vi "fpga_set.vi"(8 "error in":errorcluster, 9 "trigger  delay":u64, 10 "num samples":u64=1000, 11 "FPGA VI Reference In":refnum<k20>) -> (0 "error out":errorcluster, 3 "FPGA VI Reference Out":refnum<k20>)   [LabVIEW 2015]
doc: "Set the FPGA to wait for a trigger and aquire a specifiecf number of samples."
uses:
  <vilib>/Utility/error.llb/Error Cluster From Error Code.vi
  <vilib>/rvi/errors/niLvFpgaAdjustHostInterfaceError.vi
  <instrlib>/_niInstr/Streaming/v1/Host/Public/Start Finite Stream.vi
  <vilib>/rvi/interface/nirviReadWriteControl/nirviReadWriteControl.xnode
  <instrlib>/_niInstr/Streaming/v1/Host/niInstr Streaming v1 Host.lvlib
  NiFpgaLv.dll
  <vilib>/rvi/interface/Simulation/niFpgaSimulationCallBeginRW.vi
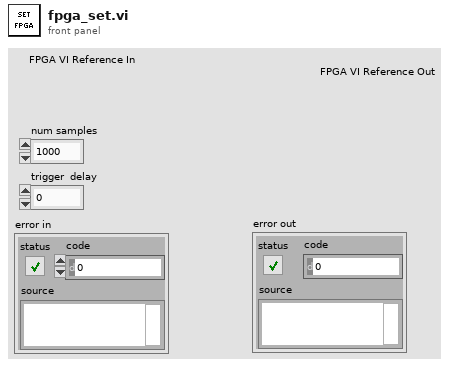
[diagram p1: front panel]
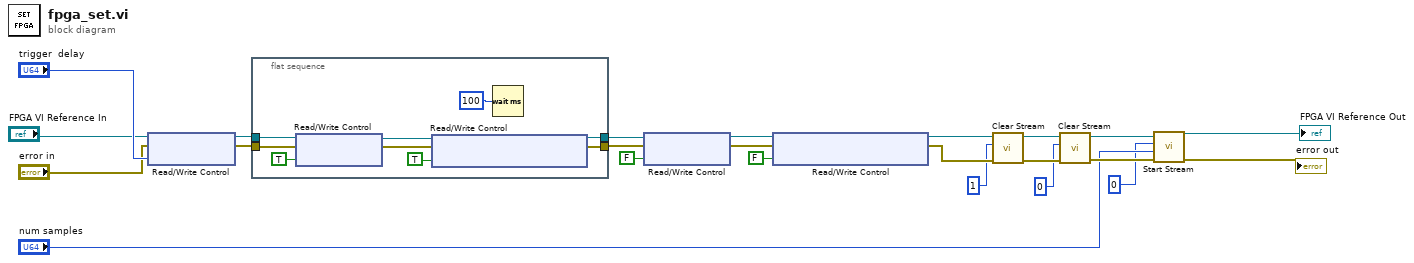
[diagram p0: block diagram]
diagram:
  n1 = xnode "Read/Write Control"("FPGA VI Reference In"="FPGA VI Reference In", "error in"="error in", "trigger  delay"="trigger  delay") -> ("FPGA VI Reference Out"=w10:refnum<k20>, "error out"=w9:errorcluster)
  n2 = flat-sequence {
    tunnel: [w30] -> w6
    tunnel: [w29] -> w7
    tunnel: w10 -> [w26]
    tunnel: w9 -> [w25]
    frame #0 {
      n3 = xnode "Read/Write Control"("FPGA VI Reference In"=w26, "error in"=w25, "Clear Trigger"=TRUE) -> ("FPGA VI Reference Out"=w28:refnum<k20>, "error out"=w27:errorcluster)
      n4 = xnode "Read/Write Control"("FPGA VI Reference In"=w28, "error in"=w27, "Reset DRAM write address"=TRUE) -> ("FPGA VI Reference Out"=w29:refnum<k20>, "error out"=w30:errorcluster)
      n5 = Wait (ms)(milliseconds to wait=u32 100) -> ()  [unwired: 1 out]
    }
  }
  n6 = xnode "Read/Write Control"("FPGA VI Reference In"=w7, "error in"=w6, "Clear Trigger"=FALSE) -> ("FPGA VI Reference Out"=w5:refnum<k20>, "error out"=w4:errorcluster)
  n7 = xnode "Read/Write Control"("FPGA VI Reference In"=w5, "error in"=w4, "Reset DRAM write address"=FALSE) -> ("FPGA VI Reference Out"=w17:refnum<k20>, "error out"=w18:errorcluster)
  n8 = call <instrlib>:"Clear Stream.vi"("error in (no error)"=w18, "stream index"=1, "refnum in"=w17) -> ("error out"=w22:errorcluster, "refnum out"=w23:refnum<k20>)  [unwired: 7 in]
  n9 = call <instrlib>:"Clear Stream.vi"("error in (no error)"=w22, "stream index"=0, "refnum in"=w23) -> ("error out"=w20:errorcluster, "refnum out"=w21:refnum<k20>)  [unwired: 7 in]
  n10 = call-poly <instrlib>:"Start Stream.vi"("error in (no error)"=w20, "num samples"="num samples", "stream index"=0, "refnum in"=w21) -> ("error out"=→"error out":errorcluster, "refnum out"=→"FPGA VI Reference Out":refnum<k20>)  [unwired: 6 in]
